vi "API GET Filter Parameters.vi"(0 "Cluster":T1={"Vin"="Vin", "R"="R", "L"="L", "C"="C", "Series"="", "Parallel"=""}, 3 "Python file path":path, 5 "docId":string="ALI00017", 9 "Select environment":enum32{"dev.", "demo.", ""}(radio), 10 "Python Version":enum32{"2.7", "3.6"}(radio), 11 "ApiToken":string, 12 "error in GET":errorcluster) -> (1 "GET RESPONSE (FromInput Names)":string, 2 "GET RESPONSE (FormInput Values)":string, 4 "Parameters Values":T2, 6 "Document Revision Id":string, 14 "GET error out":errorcluster, 15 "GET request error":errorcluster)   [LabVIEW 2019]
uses:
  Types/Parameters Values Type.ctl
  <vilib>/LVH/i3 JSON/JSON Parsing/Get Object Parameter Files/Get Object Parameter - Numeric.vi
  <vilib>/LVH/i3 JSON/JSON Parsing/Get Object Parameter Files/Get Object Parameter - Object.vi
  <vilib>/LVH/i3 JSON/JSON Parsing/Get Object Parameter Files/Get Object Parameter - String.vi
  <vilib>/LVH/i3 JSON/i3-json.lvlib
panel:
  in  "error in (no error)":errorcluster
  out "Request Status":string
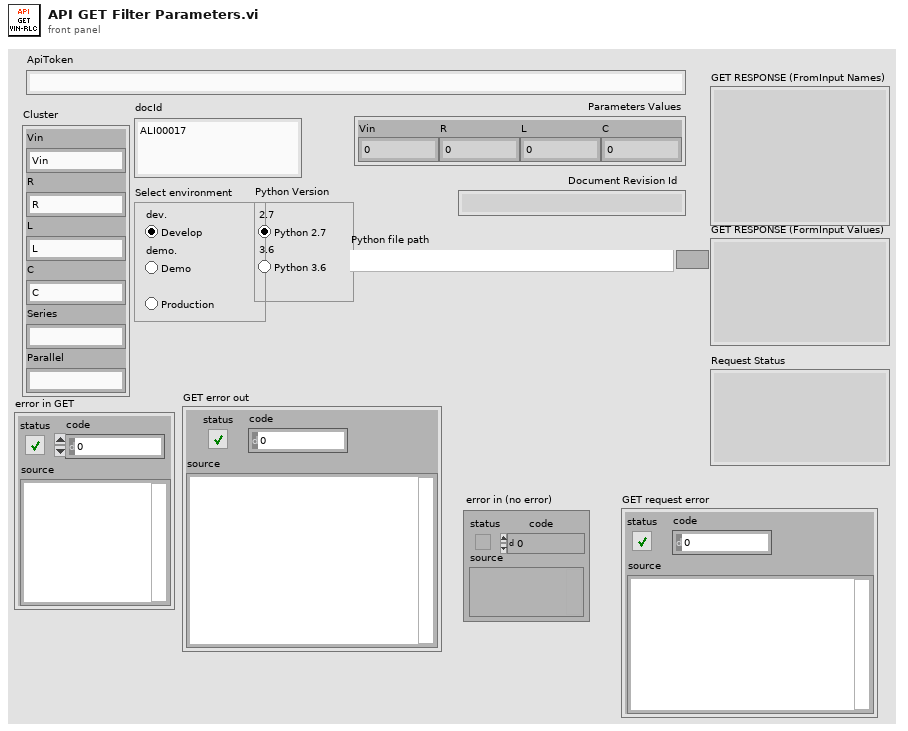
[diagram p1: front panel]
types:
  T1 = cluster{"Vin":string, "R":string, "L":string, "C":string, "Series":string, "Parallel":string}
  T2 = typedef "Parameters Values Type.ctl" = cluster{"Vin":dbl, "R":dbl, "L":dbl, "C":dbl}
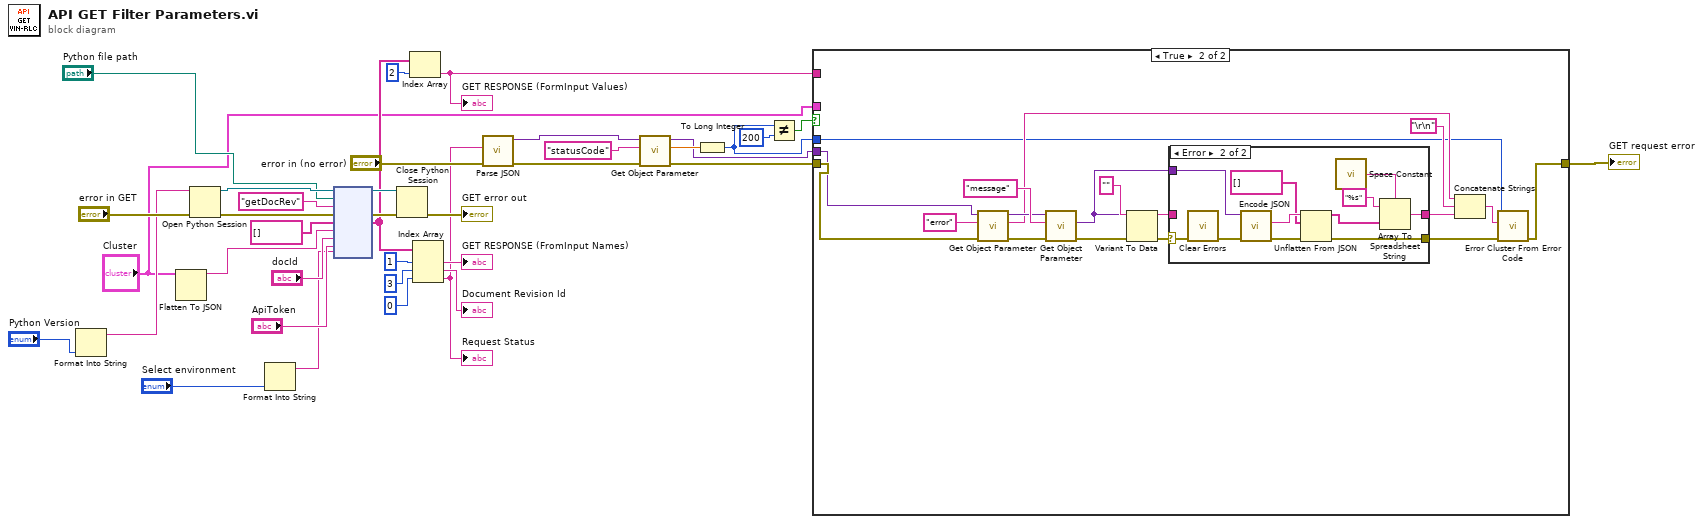
[diagram p0: block diagram]
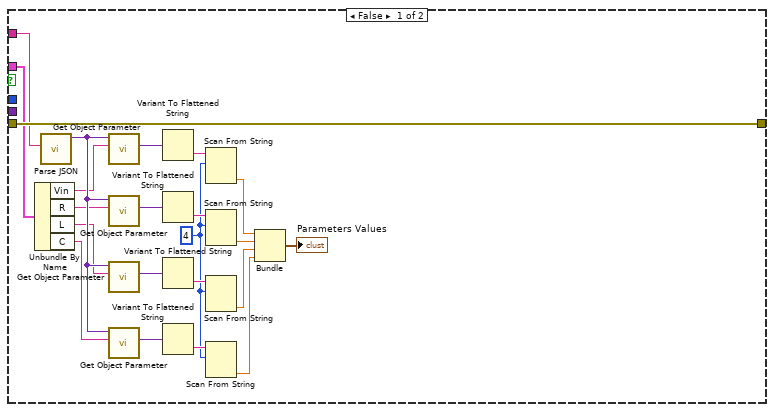
[diagram p2: hidden frame]
diagram:
  n1 = Format Into String("Python Version") -> (resulting string=w4:string)  [unwired: 3 in, 1 out]
  n2 = Flatten To JSON(anything="Cluster") -> (JSON string=w2:string)  [unwired: 2 in, 1 out]
  n3 = Open Python Session(python version=w4, 3:"error in GET") -> (session out=w35:refnum<k35>, error out=w36:errorcluster)  [unwired: 1 in]
  n4 = Format Into String("Select environment") -> (resulting string=w6:string)  [unwired: 3 in, 1 out]
  n5 = node(w35, "Python file path", "getDocRev" ("Function or Method Name"), w36, string[] [], w2, "docId", "ApiToken", w6) -> (w34:refnum<k35>, w33:errorcluster, w27:string[])  [unwired: 4 in, 2 out]
  n6 = Close Python Session(session in=w34, error in=w33) -> (11:→"GET error out":errorcluster)
  n7 = Index Array(array=w27, index=2) -> (element=w8:string)
  "GET RESPONSE (FormInput Values)" <- w8
  n8 = Index Array(array=w27, index #1=1 ("index"), index #2=3 ("index"), index #3=0 ("index")) -> (element #1=→"GET RESPONSE (FromInput Names)":string, element #2=→"Document Revision Id":string, element #3=w9:string)
  "Request Status" <- w9
  n9 = call <vilib>:"Parse JSON.vi"("error in (no error)"="error in (no error)", "JSON String"=w9) -> ("error out"=w14:errorcluster, "JSON Tree"=w16:variant)  [unwired: 6 in, 2 out]
  n10 = call-poly <vilib>:"Get Object Parameter.vi"("error in (no error)"=w14, "Parameter Name"="statusCode", "JSON Tree In (JSON Object)"=w16) -> ("error out"=w13:errorcluster, "Double Value"=w19:dbl, "JSON Tree Out Passthrough"=w12:variant)  [unwired: 5 in, 1 out]
  n11 = To Long Integer(number=w19) -> (32bit integer=w11:i32)
  n12 = Not Equal?(x=w11, y=200) -> (x != y?=w17:bool)
  n13 = case shown="True" w17 {
    tunnel: w12 -> [_ w62]
    tunnel: w13 -> [w59 w63]
    tunnel: w11 -> [_ w61]
    tunnel: [w59 w60] -> w10
    tunnel: "Cluster" -> [w39 _]
    tunnel: w8 -> [w38 _]
    frame False {
      w40 = u32 4 ("initial scan location")
      n14 = Unbundle By Name(w39) -> ("Vin"=w42:string, "R"=w43:string, "L"=w45:string, "C"=w46:string)
      n15 = call <vilib>:"Parse JSON.vi"("JSON String"=w38) -> ("JSON Tree"=w51:variant)  [unwired: 7 in, 3 out]
      n16 = call-poly <vilib>:"Get Object Parameter.vi"("Parameter Name"=w42, "JSON Tree In (JSON Object)"=w51) -> ("JSON Object"=w41:variant)  [unwired: 6 in, 3 out]
      n17 = call-poly <vilib>:"Get Object Parameter.vi"("Parameter Name"=w43, "JSON Tree In (JSON Object)"=w51) -> ("JSON Object"=w44:variant)  [unwired: 6 in, 3 out]
      n18 = call-poly <vilib>:"Get Object Parameter.vi"("Parameter Name"=w45, "JSON Tree In (JSON Object)"=w51) -> ("JSON Object"=w53:variant)  [unwired: 6 in, 3 out]
      n19 = call-poly <vilib>:"Get Object Parameter.vi"("Parameter Name"=w46, "JSON Tree In (JSON Object)"=w51) -> ("JSON Object"=w47:variant)  [unwired: 6 in, 3 out]
      n20 = Variant To Flattened String(Variant=w41) -> (data string=w48:string)  [unwired: 1 out]
      n21 = Variant To Flattened String(Variant=w44) -> (data string=w52:string)  [unwired: 1 out]
      n22 = Variant To Flattened String(Variant=w53) -> (data string=w49:string)  [unwired: 1 out]
      n23 = Variant To Flattened String(Variant=w47) -> (data string=w50:string)  [unwired: 1 out]
      n24 = Scan From String(input string=w48, initial scan location=w40) -> (output 1=w54:dbl)  [unwired: 3 in, 3 out]
      n25 = Scan From String(input string=w52, initial scan location=w40) -> (output 1=w55:dbl)  [unwired: 3 in, 3 out]
      n26 = Scan From String(input string=w49, initial scan location=w40) -> (output 1=w56:dbl)  [unwired: 3 in, 3 out]
      n27 = Scan From String(input string=w50, initial scan location=w40) -> (output 1=w57:dbl)  [unwired: 3 in, 3 out]
      n28 = Bundle(w54, w55, w56, w57) -> (→"Parameters Values":cluster{dbl, dbl, dbl, dbl})  [unwired: 1 in]
    }
    frame True {
      n29 = call-poly <vilib>:"Get Object Parameter.vi"("error in (no error)"=w63, "Parameter Name"="error", "JSON Tree In (JSON Object)"=w62) -> ("error out"=w74:errorcluster, "String Value"=w73:string, "JSON Tree Out Passthrough"=w75:variant)  [unwired: 5 in, 1 out]
      n30 = call-poly <vilib>:"Get Object Parameter.vi"("error in (no error)"=w74, "Parameter Name"="message", "JSON Tree In (JSON Object)"=w75) -> ("error out"=w69:errorcluster, "JSON Object"=w66:variant)  [unwired: 5 in, 2 out]
      n31 = Variant To Data(error in=w69, type="", Variant=w66) -> (data=w67:string, error out=w68:errorcluster)
      n32 = case shown="Error" w68 {
        selector: w68 -> [w78 w83]
        tunnel: w67 -> [w79 _]
        tunnel: [w79 w80] -> w65
        tunnel: w66 -> [_ w84]
        tunnel: [w78 w81] -> w64
        frame No Error {
        }
        frame Error {
          n33 = call <vilib>:"Clear Errors.vi"("error in (no error)"=w83) -> ("error out"=w82:errorcluster)  [unwired: 5 in, 1 out]
          n34 = call <vilib>:"Encode JSON.vi"("error in (no error)"=w82, "JSON Tree"=w84) -> ("error out"=w88:errorcluster, "String"=w87:string)  [unwired: 4 in]
          n35 = Unflatten From JSON(JSON string=w87, type and defaults=string[] [], error in (no error)=w88) -> (value=w89:string[], error out=w81:errorcluster)  [unwired: 4 in]
          n36 = call <vilib>:"Space Constant.vi"() -> ("String"=w90:string)
          n37 = Array To Spreadsheet String(delimiter (Tab)=w90, array=w89, 3:"%s" ("format string")) -> (spreadsheet string=w80:string)
        }
      }
      n38 = Concatenate Strings(w73, "\r\n", w65) -> (w72:string)
      n39 = call <vilib>:"Error Cluster From Error Code.vi"("error in (no error)"=w64, "error message (\"\")"=w72, "error code (0)"=w61) -> ("error out"=w60:errorcluster)  [unwired: 6 in]
    }
  }
  "GET request error" <- w10
